vi "Test Sampling.vi"(8 "error in (no error)":errorcluster, 11 "Instrument.Lockin in":refnum<class "Instrument.Lockin.lvclass">) -> (0 "error out":errorcluster, 3 "Instrument.Lockin out":refnum<class "Instrument.Lockin.lvclass">)   [LabVIEW 2016]
uses:
  src/Instrument.Lockin/Instrument.Lockin.lvclass
  src/Instrument.Lockin/Typedefs/Sampling.ctl
  <vilib>/addons/_JKI Toolkits/Caraya/classes/Assert/Assert Equal Value_Variant.vi
  <userlib>/_OpenG.lib/numeric/numeric.llb/Random Number Within Range - DBL__ogtk.vi
  <vilib>/addons/_JKI Toolkits/Caraya/classes/Assert/Assert Equal Value and Type_Variant.vi
  <vilib>/addons/_JKI Toolkits/Caraya/classes/Test/Test.lvclass
  <vilib>/addons/_JKI Toolkits/Caraya/classes/Assert/Assert.lvclass
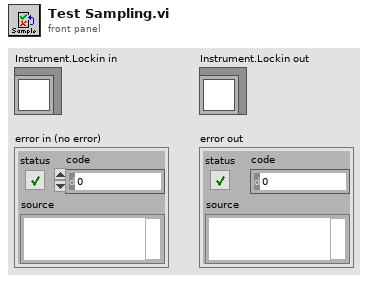
[diagram p1: front panel]
types:
  T1 = typedef "Instrument.Lockin.lvclass/Sampling.ctl" = cluster{"Fs":i32, "#s":i32}
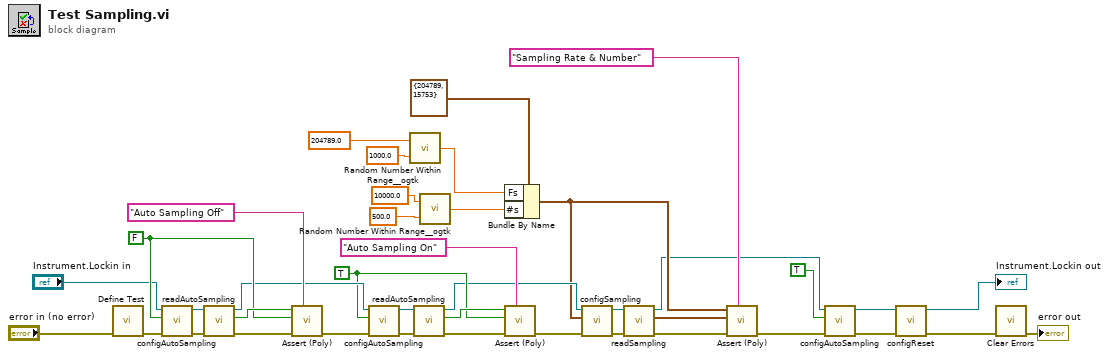
[diagram p0: block diagram]
diagram:
  w19 = TRUE ("Auto Sampling")
  w29 = FALSE ("Auto Sampling")
  n1 = call <vilib>:"Define Test.vi"("error in (no error)"="error in (no error)") -> ("error out"=w33:errorcluster)  [unwired: 10 in]
  n2 = call "configAutoSampling.vi"("error in (no error)"=w33, "Auto Sampling"=w29, "Instrument.Lockin in"="Instrument.Lockin in") -> ("error out"=w32:errorcluster, "Instrument.Lockin out"=w31:refnum<class "Instrument.Lockin.lvclass">)  [unwired: 7 in]
  n3 = call "readAutoSampling.vi"("error in (no error)"=w32, "Instrument.Lockin in"=w31) -> ("error out"=w28:errorcluster, "Auto Sampling"=w30:bool, "Instrument.Lockin out"=w21:refnum<class "Instrument.Lockin.lvclass">)  [unwired: 7 in]
  n4 = call-poly <vilib>:"Assert (Poly).vi"("Label"="Auto Sampling Off", "error in (no error)"=w28, "Y"=w29, "X"=w30) -> ("error out"=w20:errorcluster)  [unwired: 7 in]
  n5 = call "configAutoSampling.vi"("error in (no error)"=w20, "Auto Sampling"=w19, "Instrument.Lockin in"=w21) -> ("error out"=w22:errorcluster, "Instrument.Lockin out"=w23:refnum<class "Instrument.Lockin.lvclass">)  [unwired: 7 in]
  n6 = call-poly <userlib>:"Random Number Within Range__ogtk.vi"("High"=204789.0, "Low"=1000.0) -> ("Random Number"=w11:dbl)  [unwired: 3 in]
  n7 = call "readAutoSampling.vi"("error in (no error)"=w22, "Instrument.Lockin in"=w23) -> ("error out"=w25:errorcluster, "Auto Sampling"=w24:bool, "Instrument.Lockin out"=w17:refnum<class "Instrument.Lockin.lvclass">)  [unwired: 7 in]
  n8 = call-poly <userlib>:"Random Number Within Range__ogtk.vi"("High"=10000.0, "Low"=500.0) -> ("Random Number"=w8:dbl)  [unwired: 3 in]
  n9 = Bundle By Name(cluster=T1 {"Fs"=204789, "#s"=15753} ("Sampling"), "Fs"=w11, "#s"=w8) -> (w12:T1)
  n10 = call-poly <vilib>:"Assert (Poly).vi"("Label"="Auto Sampling On", "error in (no error)"=w25, "Y"=w19, "X"=w24) -> ("error out"=w16:errorcluster)  [unwired: 7 in]
  n11 = call "configSampling.vi"("error in (no error)"=w16, "Sampling"=w12, "Instrument.Lockin in"=w17) -> ("error out"=w36:errorcluster, "Instrument.Lockin out"=w35:refnum<class "Instrument.Lockin.lvclass">)  [unwired: 7 in]
  n12 = call "readSampling.vi"("error in (no error)"=w36, "Instrument.Lockin in"=w35) -> ("error out"=w38:errorcluster, "sampling"=w39:T1, "Instrument.Lockin out"=w6:refnum<class "Instrument.Lockin.lvclass">)  [unwired: 7 in]
  n13 = call-poly <vilib>:"Assert (Poly).vi"("Label"="Sampling Rate & Number", "error in (no error)"=w38, "Y"=w39, "X"=w12) -> ("error out"=w5:errorcluster)  [unwired: 7 in]
  n14 = call "configAutoSampling.vi"("error in (no error)"=w5, "Auto Sampling"=TRUE, "Instrument.Lockin in"=w6) -> ("error out"=w4:errorcluster, "Instrument.Lockin out"=w2:refnum<class "Instrument.Lockin.lvclass">)  [unwired: 7 in]
  n15 = call "configReset.vi"("error in (no error)"=w4, "Instrument.Lockin in"=w2) -> ("error out"=w3:errorcluster, "Instrument.Lockin out"=→"Instrument.Lockin out":refnum<class "Instrument.Lockin.lvclass">)  [unwired: 8 in]
  n16 = call <vilib>:"Clear Errors.vi"("error in (no error)"=w3) -> ("error out"=→"error out":errorcluster)  [unwired: 5 in, 1 out]
